vi "MT Generate FSK Synchronization Parameters (bit array).vi"(0 "FSK system parameters":T1={"samples per symbol (16)"=16, "symbol map"=[], "symbol phase continuity"=enum."continuous"} {"symbol map" format="%.2f"}, 5 "sync bits":i8[](array[numeric]), 11 "error in (no error)":errorcluster, 12 "expected sync location (symbols)":i32=-1, 13 "sync location uncertainty (symbols)":i32=10, 14 "sync indent (symbols)":i32) -> (4 "FSK synchronization parameters":T2 {"sync sequence" format="%.2f"}, 15 "error out":errorcluster)   [LabVIEW 2020, in "niDMT.lvlib"]
doc: "This polymorphic instance generates synchronization parameters for FSK demodulation using a synchronization sequence directly represented by the <B>sync bits</B> input array."
uses:
  <vilib>/addons/Modulation/niDMT.lvlib
  <vilib>/addons/Modulation/niAMT.lvlib
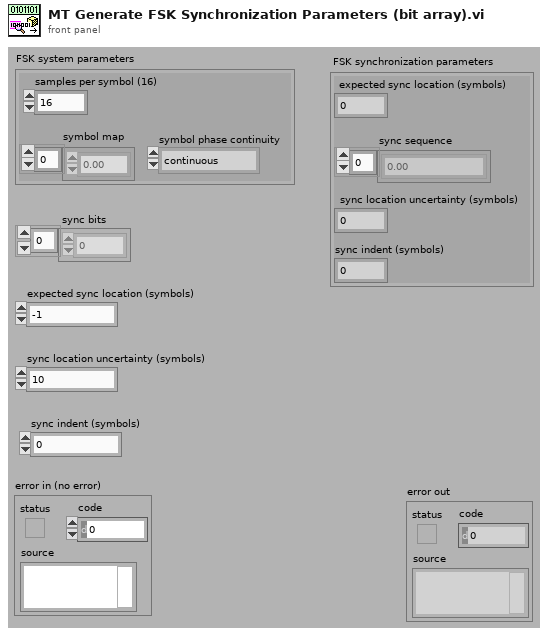
[diagram p1: front panel]
types:
  T1 = cluster{"samples per symbol (16)":i32, "symbol map":dbl[], "symbol phase continuity":enum16{"continuous", "discontinuous"}}
  T2 = cluster{"expected sync location (symbols)":i32, "sync sequence":cdb[], "sync location uncertainty (symbols)":i32, "sync indent (symbols)":i32}
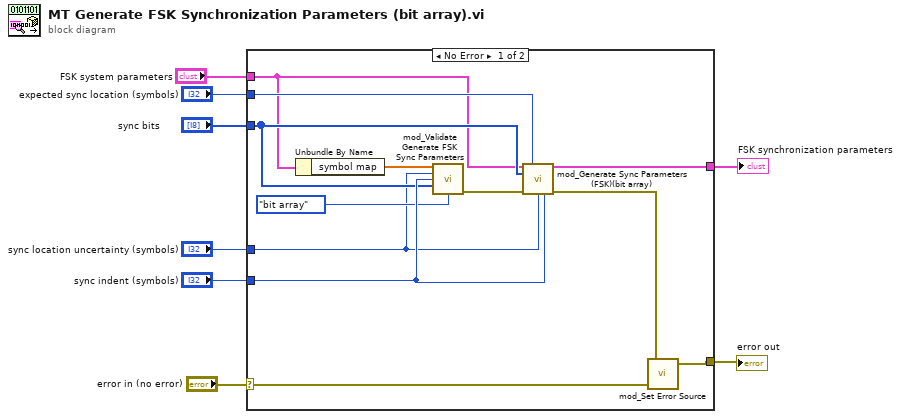
[diagram p0: block diagram]
diagram:
  n1 = case shown="No Error" "error in (no error)" {
    selector: "error in (no error)" -> [w19 w21]
    tunnel: "FSK system parameters" -> [w10 _]
    tunnel: "expected sync location (symbols)" -> [w17 _]
    tunnel: "sync location uncertainty (symbols)" -> [w9 _]
    tunnel: "sync indent (symbols)" -> [w13 _]
    tunnel: "sync bits" -> [w12 _]
    tunnel: [w20 w21] -> w2
    tunnel: [w18 _] -> w1
    frame No Error {
      n2 = Unbundle By Name(w10) -> ("symbol map"=w15:dbl[])
      n3 = call <vilib>:"mod_Validate Generate FSK Sync Parameters.vi"("symbol map"=w15, "sync location uncertainty (symbols)"=w9, "sync indent (symbols)"=w13, "sync bits"=w12, "sync bits specification"=enum16{"bit array", "number array", "number"}."bit array") -> ("error out"=w14:errorcluster)  [unwired: 2 in, 8 out]
      n4 = call <vilib>:"mod_Generate Sync Parameters (FSK)(bit array).vi"("FSK system parameters"=w10, "sync bits"=w12, "error in (no error)"=w14, "expected sync location (symbols)"=w17, "sync location uncertainty (symbols)"=w9, "sync indent (symbols)"=w13) -> ("FSK synchronization parameters"=w18:T2, "error out"=w16:errorcluster)  [unwired: 8 out]
      n5 = call <vilib>:"mod_Set Error Source.vi"("initial error in (no error)"=w19, "final error in (no error)"=w16) -> ("error out"=w20:errorcluster)  [unwired: 3 out]
    }
    frame Error {
    }
  }
  "FSK synchronization parameters" <- w1
  "error out" <- w2
